vi "Create Index to Methods.vi"(8 "error in":errorcluster, 10 "versions":i32[](array[numeric]), 11 "Method Names":string[](array[string])) -> (0 "error out":errorcluster)   [LabVIEW 2012]
uses:
  Folders.ctl
  Design Server.lvlib
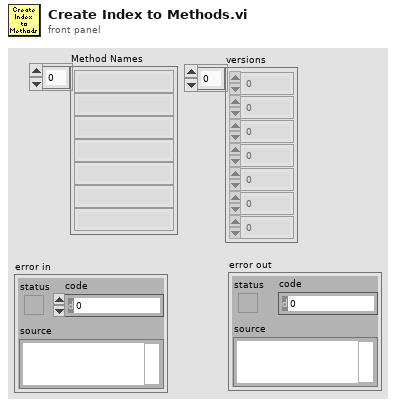
[diagram p1: front panel]
types:
  T1 = enum16{"open", "replace", "create", "open or create", "replace or create", "replace or create with confirmation"}
  T2 = typedef "Design Server.lvlib/Folders.ctl" = enum16{"MathcadMethods", "RequestedDesigns", "CompletedDesigns", "MathcadCode", "CollabnetSVN.exe"}
  T3 = typedef "Method.ctl" = cluster{"Title":string, "About":string, "Input Parameters":cluster{"Description":string, "Name":string, "Min":string, "Max":string, "Default":string, "Units":string, "Increment":string, "Stock designs":string[]}[], "AutoCAD drawings":cluster{"File Name":string, "AC Variables":string[]}[], "Stock file names":string[], "Publish files":string[], "Display images":string[]}
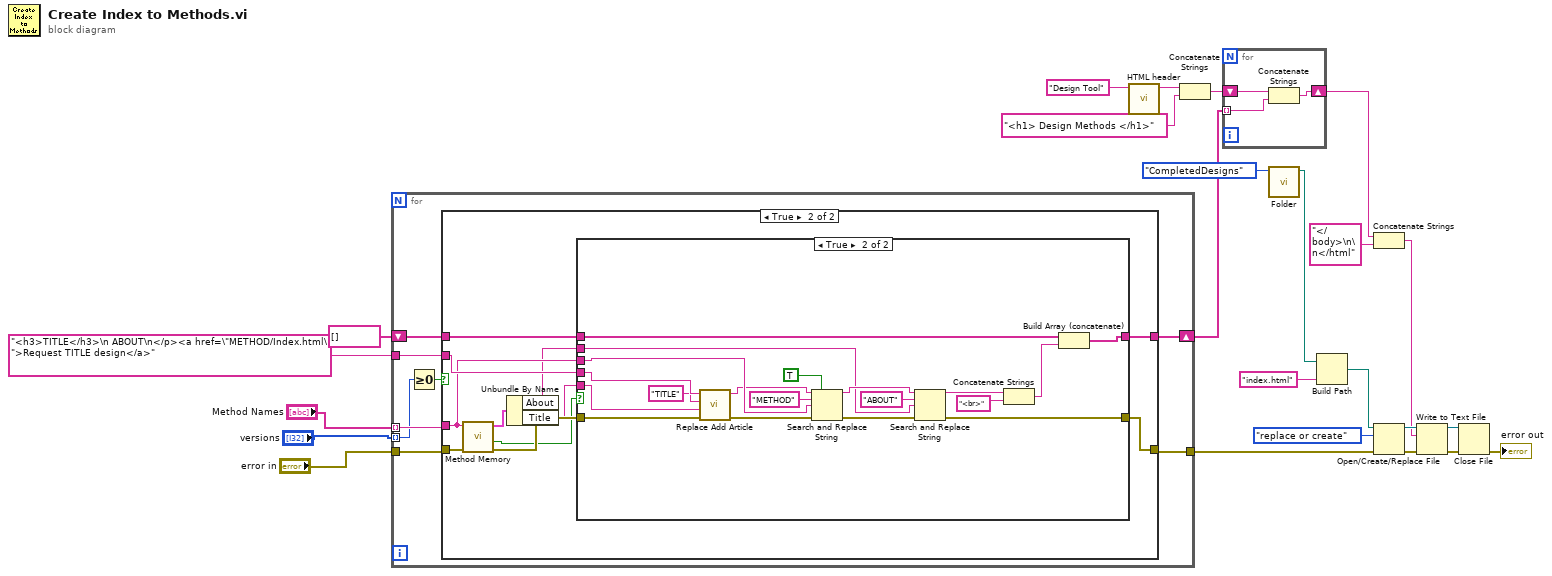
[diagram p0: block diagram]
diagram:
  n1 = for {
    tunnel: "Method Names" -> [w27] mode=indexing
    tunnel: "error in" -> [w32]
    tunnel: "<h3>TITLE</h3>\n ABOUT\n</p><a href=\"METHOD/Index.html\">Request TITLE design</a>" -> [w31]
    tunnel: [w30] -> w5
    shift-right: [w29] -> w8
    shift-left: string[] [] -> [w28]
    tunnel: "versions" -> [w25] mode=indexing
    n2 = Greater Or Equal To 0?(x=w25) -> (x >= 0?=w26:bool)
    n3 = case shown="True" w26 {
      tunnel: w32 -> [w34 w45]
      tunnel: w31 -> [_ w44]
      tunnel: [w34 w42] -> w30
      tunnel: [w33 w41] -> w29
      tunnel: w28 -> [w33 w40]
      tunnel: w27 -> [_ w39]
      frame False {
      }
      frame True {
        n4 = call "Method Memory.vi"("error in"=w45, "Method Name"=w39) -> ("error out"=w43:errorcluster, "method exists?"=w38:bool, "Method Out"=w37:T3)  [unwired: 7 in]
        n5 = Unbundle By Name(w37) -> ("About"=w35:string, "Title"=w36:string)
        n6 = case shown="True" w38 {
          tunnel: w44 -> [_ w52]
          tunnel: w43 -> [w47 w54]
          tunnel: w39 -> [_ w65]
          tunnel: w35 -> [_ w48]
          tunnel: [w47 w59] -> w42
          tunnel: [w46 w57] -> w41
          tunnel: w40 -> [w46 w56]
          tunnel: w36 -> [_ w50]
          frame False {
          }
          frame True {
            n7 = call "Replace Add Article.vi"("error in (no error)"=w54, "Replacement"=w50, "KEY"="TITLE" ("search string"), "Input String"=w52) -> ("error out"=w55:errorcluster, "result string"=w53:string)  [unwired: 6 in]
            n8 = Search and Replace String(replace all?=TRUE ("replace all? (F)"), input string=w53, search string="METHOD", replace string=w65, error in=w55) -> (result string=w63:string, error out=w64:errorcluster)  [unwired: 3 in, 2 out]
            n9 = Search and Replace String(input string=w63, search string="ABOUT", replace string=w48, error in=w64) -> (result string=w61:string, error out=w59:errorcluster)  [unwired: 4 in, 2 out]
            n10 = Concatenate Strings(w61, "<br>" ("string")) -> (w49:string)
            n11 = Build Array (concatenate)(w56, w49) -> (w57:string[])
          }
        }
      }
    }
  }
  n12 = call "HTML header.vi"("Title"="Design Tool") -> ("HTML header"=w12:string)  [unwired: 10 in]
  n13 = Concatenate Strings(w12, "<h1> Design Methods </h1>") -> (w9:string)
  n14 = for {
    tunnel: w8 -> [w67] mode=indexing
    shift-right: [w69] -> w14
    shift-left: w9 -> [w68]
    n15 = Concatenate Strings(w68, w67) -> (w69:string)
  }
  n16 = call "Folder.vi"("Folders"=Folders."CompletedDesigns") -> ("FolderPath"=w23:path)  [unwired: 8 in, 2 out]
  n17 = Build Path(base path=w23, name or relative path="index.html") -> (appended path=w21:path)
  n18 = Concatenate Strings(w14, "</body>\n\n</html") -> (w6:string)
  n19 = Open/Create/Replace File(file path (use dialog)=w21, error in=w5, operation (0:open)=T1."replace or create") -> (refnum out=w16:refnum<file>, error out=w19:errorcluster)  [unwired: 3 in, 1 out]
  n20 = Write to Text File(file (use dialog)=w16, text=w6, error in=w19) -> (refnum out=w17:refnum<file>, error out=w18:errorcluster)  [unwired: 1 in, 1 out]
  n21 = Close File(refnum=w17, error in=w18) -> (error out=→"error out":errorcluster)  [unwired: 1 out]
